vi "Configure Bus Controller.vi"(8 "error in (no error)":errorcluster) -> (0 "error out":errorcluster, 3 "Bus Controller":refnum<class "Bus Controller.lvclass">)   [LabVIEW 2020, in "BCI-1553 RealTime API Examples.lvlib"]
uses:
  BCI-1553 RealTime API Examples.lvlib
  src/RealTime/Bus Controller/Bus Controller.lvclass
  src/RealTime/Bus Controller/TypeDefs/Bus Controller Configuration.ctl
  src/RealTime/Bus Controller/TypeDefs/Bus Controller Timeout.ctl
  src/RealTime/Frames & Messages/Major Frame/Major Frame.lvclass
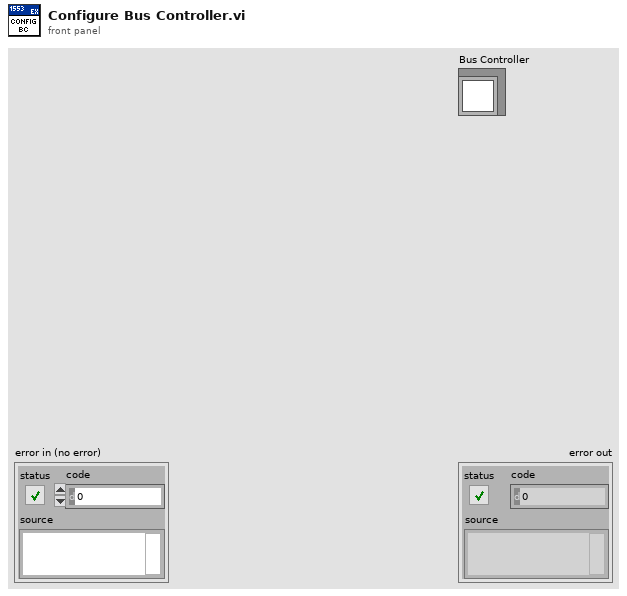
[diagram p1: front panel]
types:
  T1 = typedef "BCI-1553 API.lvlib/Bus Controller.lvclass/Bus Controller Timeout.ctl" = enum16{"17us", "22us", "60us", "140us"}
  T2 = typedef "BCI-1553 API.lvlib/Bus Controller.lvclass/Bus Controller Configuration.ctl" = cluster{"Timeout":T1, "BC Retry":bool, "BC Second Retry":bool, "BC Retry Alt Bus":bool, "BC Second Retry Alt Bus":bool, "BC Retry on Status Bit":bool, "Msg Error No Data Valid":bool, "Busy Status No Data Valid":bool, "Msg Gap Timer":bool, "Watchdog Timer":bool, "Time Tag Sync":bool, "Even Time Tag Sync":bool, "Gap Check":bool, "Broadcast Mask Enable":bool}
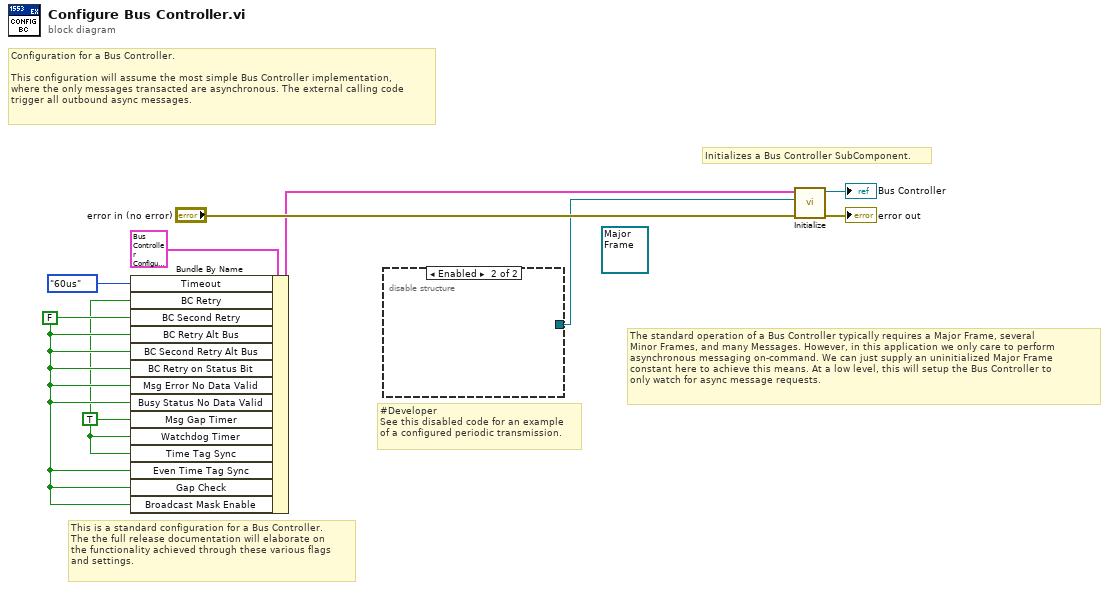
[diagram p0: block diagram]
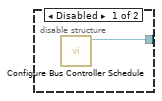
[diagram p2: hidden frame]
diagram:
  w2 = TRUE ("Msg Gap Timer")
  w3 = FALSE ("BC Retry")
  (unwired) refnum<class "Major Frame.lvclass"> refnum ("Major Frame")
  # "#Developer\nSee this disabled code for an example\nof a configured periodic transmission."
  # "Initializes a Bus Controller SubComponent."
  # "This is a standard configuration for a Bus Controller.\nThe the full release documentation will elaborate on\nthe functionality achieved through these various flags\nand settings."
  # "The standard operation of a Bus Controller typically requires a Major Frame, several \nMinor Frames, and many Messages. However, in this application we only care to perform\nasynchronous messaging on-command. We can just supply an uninitialized Major Frame\nconstant here to achieve this means. At a low level, this will setup the Bus Controller to\nonly watch for async message requests."
  # "Configuration for a Bus Controller.\n\nThis configuration will assume the most simple Bus Controller implementation,\nwhere the only messages transacted are asynchronous. The external calling code\ntrigger all outbound async messages."
  n1 = Bundle By Name(cluster=T2 {"Timeout"=enum."17us", "BC Retry"=FALSE, "BC Second Retry"=FALSE, "BC Retry Alt Bus"=FALSE, "BC Second Retry Alt Bus"=FALSE, "BC Retry on Status Bit"=FALSE, "Msg Error No Data Valid"=FALSE, "Busy Status No Data Valid"=FALSE, "Msg Gap Timer"=FALSE, "Watchdog Timer"=FALSE, "Time Tag Sync"=FALSE, "Even Time Tag Sync"=FALSE, "Gap Check"=FALSE, "Broadcast Mask Enable"=FALSE} ("Configuration"), "Timeout"=Bus_Controller_Timeout."60us", "BC Retry"=w2, "BC Second Retry"=w3, "BC Retry Alt Bus"=w3, "BC Second Retry Alt Bus"=w3, "BC Retry on Status Bit"=w3, "Msg Error No Data Valid"=w3, "Busy Status No Data Valid"=w3, "Msg Gap Timer"=w2, "Watchdog Timer"=w2, "Time Tag Sync"=w2, "Even Time Tag Sync"=w3, "Gap Check"=w3, "Broadcast Mask Enable"=w3) -> (w5:T2)
  n2 = disable-structure shown="Enabled" {
    disable-tunnel: [w10 _] -> w1
    frame Disabled {
      n3 = call "Configure Bus Controller Schedule.vi"() -> ("Major Frame (Scheduled)"=w10:refnum<class "Major Frame.lvclass">)  [unwired: 10 in, 1 out]
    }
    frame Enabled {
    }
  }
  n4 = call "Initialize.vi"("error in (no error)"="error in (no error)", "Major Frame"=w1, "Configuration"=w5) -> ("error out"=→"error out":errorcluster, "Bus Controller out"=→"Bus Controller":refnum<class "Bus Controller.lvclass">)  [unwired: 7 in]
